vi "认识比较.vi"() -> ()   [LabVIEW 2018]
panel:
  out "温度情况":string
  in  "停止":bool
  out "报警":bool
  in  "设定值":dbl
  out "温度计":dbl(slide) scale=0.0..100.0
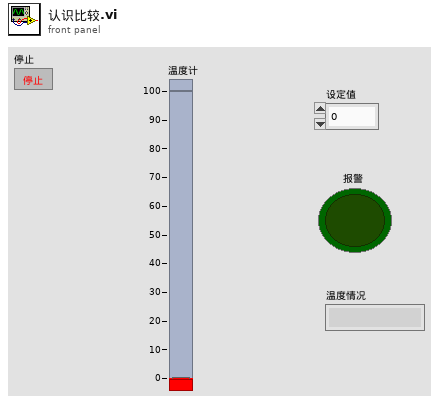
[diagram p1: front panel]
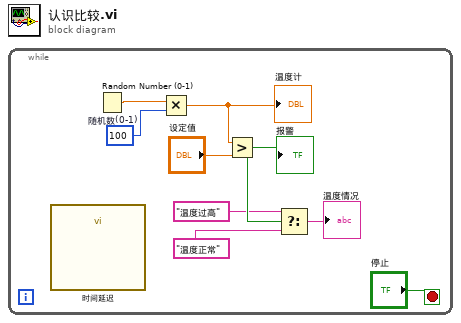
[diagram p0: block diagram]
diagram:
  n1 = while {
    stop <- "停止" stop-if-true
    n2 = call "时间延迟"() -> ()  [unwired: 11 in, 1 out]
    n3 = Random Number (0-1) "随机数(0-1)"() -> (number: 0 to 1=w9:dbl)
    n4 = Multiply(x=w9, y=100) -> (x*y=w7:dbl)
    "温度计" <- w7
    n5 = Greater?(x=w7, y="设定值") -> (0:w4:bool)
    "报警" <- w4
    n6 = Select(t="温度过高", s=w4, f="温度正常") -> (s? t:f=→"温度情况":string)
  }
